vi "Set State_Measure SMU_W Delay Control.vi"(5 "Delay Time (s)":dbl=0.001 format="%#_13p", 6 "SMU Settings":T2={"Level"=0.01, "Level Range"=0.1, "Limit"=1.0, "Limit Range"=6.0, "Sense"=1009} {"Sense" items=["Local"=1008, "Remote"=1009]}, 7 "script name":string, 8 "error in (no error)":errorcluster, 9 "Published Data Ids":string[](array[string]), 10 "Pins":string[](array[string])=["VDD"], 11 "Semiconductor Module Context":T3) -> (0 "error Out":errorcluster)   [LabVIEW 2013]
uses:
  <vilib>/NI_TestStand_SemiconductorModule/NI_TestStand_Semiconductor_Module.lvlibp/PinMap/General/SemiconductorModuleContext.ctl
  <instrlib>/niDCPower/nidcpower.llb/niDCPower Sense.ctl
  <instrlib>/niHSDIO/niHSDIO.llb/niHSDIO_ctl Trigger Script - trigID Values (Ring).ctl
  <vilib>/NI_TestStand_SemiconductorModule/NI_TestStand_Semiconductor_Module.lvlibp
panel:
  out "R Array":dbl[][](array[numeric]) format="%#_6p"
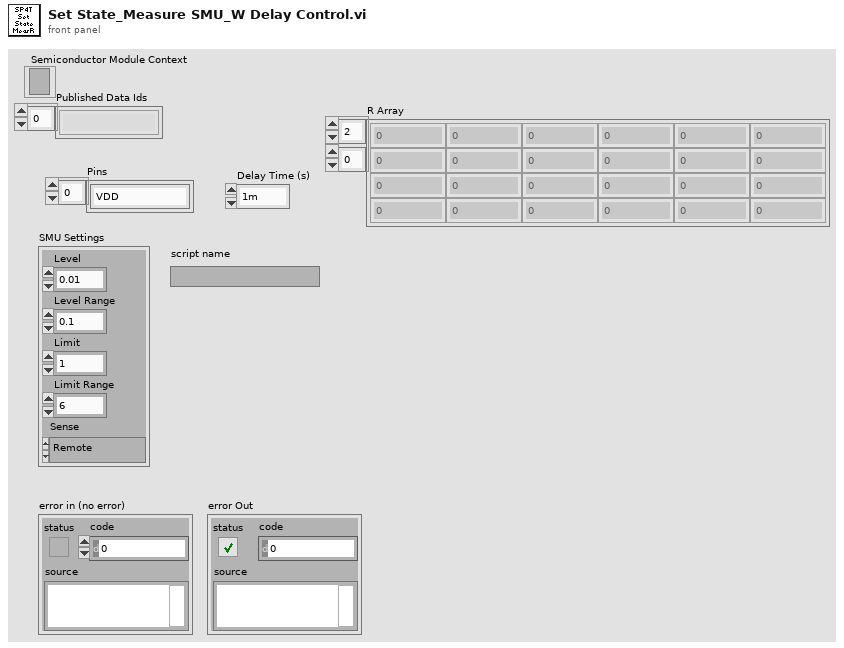
[diagram p1: front panel]
types:
  T1 = typedef "niDCPower Sense.ctl" = i32
  T2 = cluster{"Level":dbl, "Level Range":dbl, "Limit":dbl, "Limit Range":dbl, "Sense":T1}
  T3 = typedef "NI_TestStand_Semiconductor_Module.lvlibp/SemiconductorModuleContext.ctl" = refnum<k7>
  T4 = typedef "niHSDIO_ctl Trigger Script - trigID Values (Ring).ctl" = string
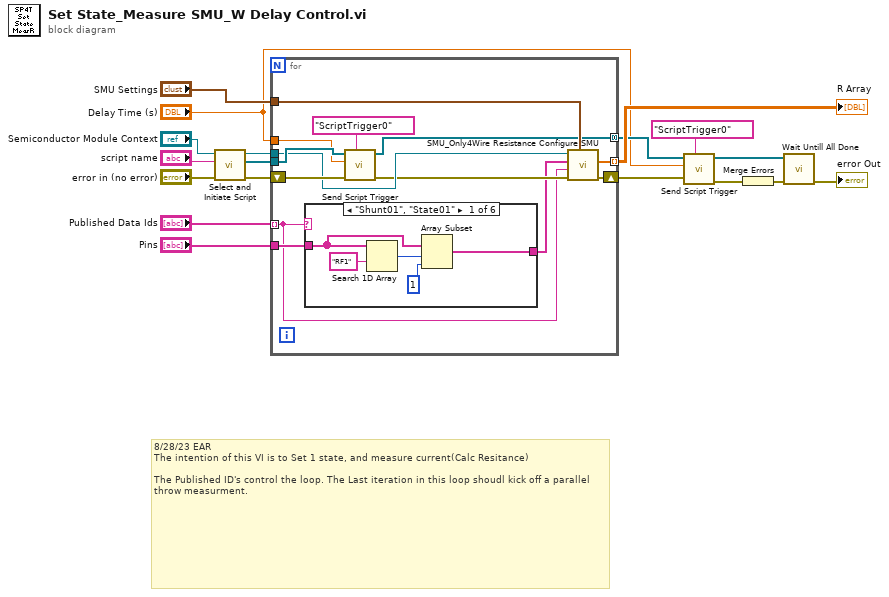
[diagram p0: block diagram]
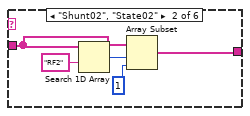
[diagram p2: hidden frame]
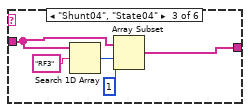
[diagram p3: hidden frame]
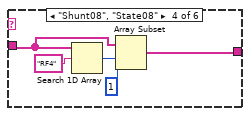
[diagram p4: hidden frame]
diagram:
  # "8/28/23 EAR\nThe intention of this VI is to Set 1 state, and measure current(Calc Resitance)\n\nThe Published ID's control the loop. The Last iteration in this loop shoudl kick off a parallel throw measurment."
  n1 = call "Select and Initiate Script.vi"("error in (no error)"="error in (no error)", "script name"="script name", "Semiconductor Module Context"="Semiconductor Module Context") -> ("error out"=w16:errorcluster, "HSDIO GEN Sessions Out"=w15:refnum<k15>[], "Semiconductor Module Context Out"=w12:T3)  [unwired: 6 in]
  n2 = for {
    tunnel: w15 -> [w29]
    tunnel: "SMU Settings" -> [w28]
    tunnel: w12 -> [w27]
    tunnel: "Published Data Ids" -> [w21] mode=indexing
    tunnel: "Pins" -> [w23]
    tunnel: [w24] -> w9 mode=indexing
    tunnel: [w20] -> w3 mode=concatenating
    shift-right: [w31] -> w4
    shift-left: w16 -> [w30]
    tunnel: "Delay Time (s)" -> [w19]
    n3 = case shown="\"Shunt01\", \"State01\"" w21 {
      tunnel: w23 -> [w35 w38 w45 w47 w52 w53]
      tunnel: [w34 w37 w44 w48 w52 w53] -> w22
      frame "Shunt01", "State01" {
        n4 = Search 1D Array(1D array=w35, element="RF1") -> (index of element=w33:i32)  [unwired: 1 in]
        n5 = Array Subset(array=w35, index=w33, length=1) -> (w34:string[])
      }
      frame "Shunt02", "State02" {
        n6 = Search 1D Array(1D array=w38, element="RF2") -> (index of element=w40:i32)  [unwired: 1 in]
        n7 = Array Subset(array=w38, index=w40, length=1) -> (w37:string[])
      }
      frame "Shunt04", "State04" {
        n8 = Search 1D Array(1D array=w45, element="RF3") -> (index of element=w43:i32)  [unwired: 1 in]
        n9 = Array Subset(array=w45, index=w43, length=1) -> (w44:string[])
      }
      frame "Shunt08", "State08" {
        n10 = Search 1D Array(1D array=w47, element="RF4") -> (index of element=w50:i32)  [unwired: 1 in]
        n11 = Array Subset(array=w47, index=w50, length=1) -> (w48:string[])
      }
      frame "Shunt15", "State15" {
      }
      frame "Shunt00", "State00", Default {
      }
    }
    n12 = call "Send Script Trigger.vi"("trigger id (script trigger 0)"=T4 "ScriptTrigger0", "error in (no error)"=w30, "Delay Time (s)"=w19, "HSDIO Sessions In"=w29) -> ("error out"=w25:errorcluster, "HSDIO Sessions Out"=w20:refnum<k15>[])  [unwired: 6 in]
    n13 = call "SMU_Only4Wire Resistance Configure SMU.vi"("SMU Settings"=w28, "error in (no error)"=w25, "Published Data Id"=w21, "Pins"=w22, "Semiconductor Module Context"=w27) -> ("error Out"=w31:errorcluster, "R Array"=w24:dbl[])  [unwired: 4 in, 1 out]
  }
  "R Array" <- w9
  n14 = call "Send Script Trigger.vi"("trigger id (script trigger 0)"=T4 "ScriptTrigger0", "error in (no error)"=w4, "Delay Time (s)"="Delay Time (s)", "HSDIO Sessions In"=w3) -> ("error out"=w5:errorcluster, "HSDIO Sessions Out"=w2:refnum<k15>[])  [unwired: 6 in]
  n15 = Merge Errors(w5) -> (w8:errorcluster)
  n16 = call "Wait Untill All Done.vi"("error in (no error)"=w8, "HSDIO Sessions In"=w2) -> ("error out"=→"error Out":errorcluster)  [unwired: 8 in, 1 out]
